vi "Ramp PSU to Zero.vi"(8 "error in (no error)":errorcluster, 11 "Instrument.Oxford1820 in":refnum<class "Instrument.Oxford1820.lvclass">) -> (0 "error out":errorcluster, 3 "Instrument.Oxford1820 out":refnum<class "Instrument.Oxford1820.lvclass">)   [LabVIEW 2016]
uses:
  Instrument.Oxford1820.lvclass
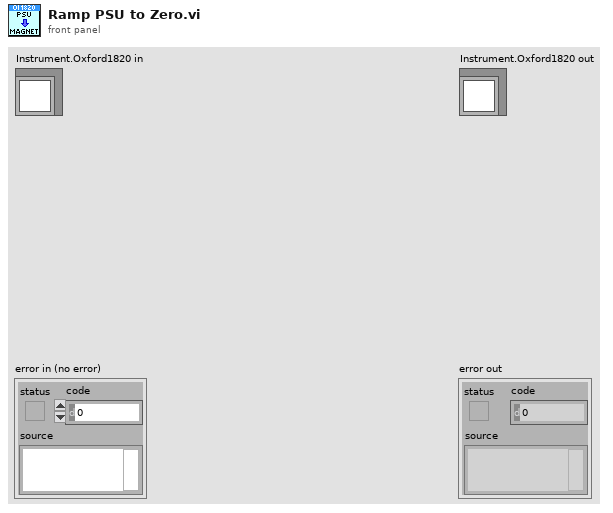
[diagram p1: front panel]
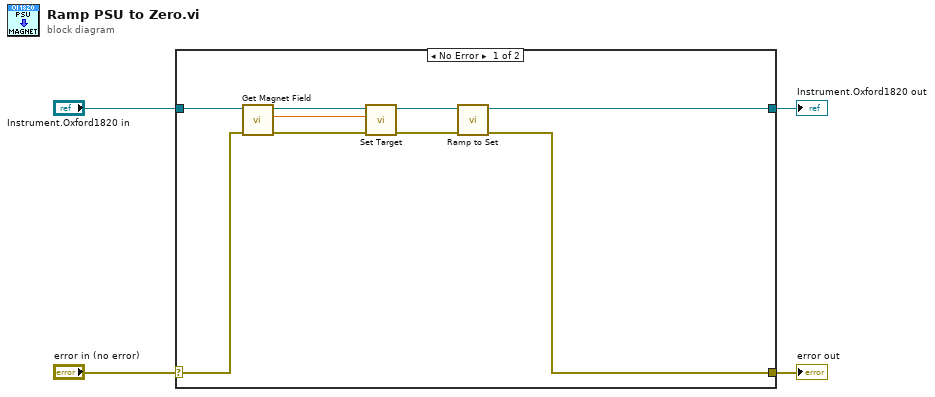
[diagram p0: block diagram]
diagram:
  n1 = case shown="No Error" "error in (no error)" {
    selector: "error in (no error)" -> [w6 w15]
    tunnel: [w5 w15] -> w3
    tunnel: [w7 w14] -> w1
    tunnel: "Instrument.Oxford1820 in" -> [w12 w14]
    frame No Error {
      n2 = call-dynamic "Get Magnet Field.vi"("error in (no error)"=w6, "Instrument.Oxford1820 in"=w12) -> ("error out"=w10:errorcluster, "B Field (T)"=w13:dbl, "Instrument.Oxford1820 out"=w11:refnum<class "Instrument.Oxford1820.lvclass">)  [unwired: 5 in, 2 out]
      n3 = call-dynamic "Set Target.vi"("error in (no error)"=w10, "Target Field (T)"=w13, "Instrument.Oxford1820 in"=w11) -> ("error out"=w8:errorcluster, "Instrument.Oxford1820 out"=w9:refnum<class "Instrument.Oxford1820.lvclass">)  [unwired: 7 in]
      n4 = call-dynamic "Ramp to Set.vi"("error in (no error)"=w8, "Instrument.Oxford1820 in"=w9) -> ("error out"=w5:errorcluster, "Instrument.Oxford1820 out"=w7:refnum<class "Instrument.Oxford1820.lvclass">)  [unwired: 8 in]
    }
    frame Error {
    }
  }
  "error out" <- w3
  "Instrument.Oxford1820 out" <- w1
